vi "Path_Support Directory.vi"() -> (3 "Support Directory":path)   [LabVIEW 2023]
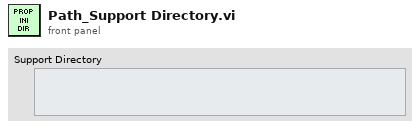
[diagram p1: front panel]
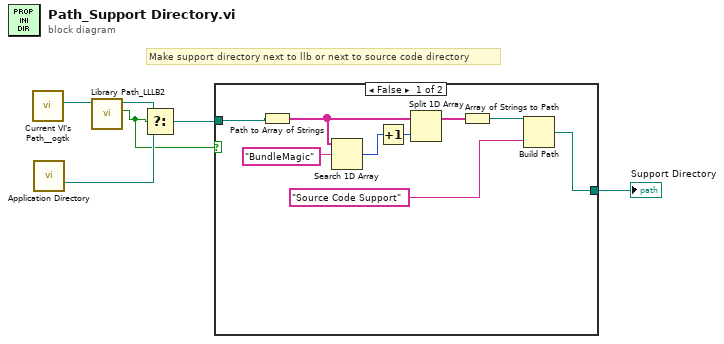
[diagram p0: block diagram]
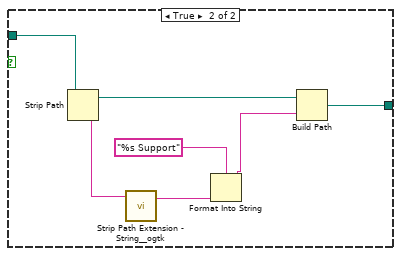
[diagram p2: hidden frame]
diagram:
  # "Make support directory next to llb or next to source code directory"
  n1 = call <userlib>:"Current VI's Path__ogtk.vi"() -> ("Current VI's Path (+ Relative)"=w3:path)  [unwired: 1 in]
  n2 = call <vilib>:"Application Directory.vi"() -> ("Application Directory"=w5:path)
  n3 = call "Library Path_LLLB2.vi"("File Path"=w3) -> ("Is in llb?"=w1:bool, "llb path"=w2:path)  [unwired: 9 in]
  n4 = Select(t=w2, s=w1, f=w5) -> (s? t:f=w4:path)
  n5 = case shown="False" w1 {
    tunnel: [w8 w17] -> w6
    tunnel: w4 -> [w15 w16]
    frame False {
      n6 = Path to Array of Strings(0:w15) -> (2:w13:string[])  [unwired: 1 out]
      n7 = Search 1D Array(1D array=w13, element="BundleMagic") -> (index of element=w12:i32)  [unwired: 1 in]
      n8 = Increment(x=w12) -> (x+1=w7:i32)
      n9 = Split 1D Array(array=w13, index=w7) -> (first subarray=w11:string[])  [unwired: 1 out]
      n10 = Array of Strings to Path(0:w11) -> (2:w10:path)  [unwired: 1 in]
      n11 = Build Path(base path=w10, name or relative path="Source Code Support" ("element")) -> (appended path=w8:path)
    }
    frame True {
      n12 = Strip Path(path=w16) -> (stripped path=w22:path, name=w21:string)
      n13 = call <userlib>:"Strip Path Extension - String__ogtk.vi"("path"=w21) -> ("root"=w20:string)  [unwired: 1 out]
      n14 = Format Into String(format string="%s Support", w20) -> (resulting string=w18:string)  [unwired: 2 in, 1 out]
      n15 = Build Path(base path=w22, name or relative path=w18) -> (appended path=w17:path)
    }
  }
  "Support Directory" <- w6
